vi "FFID_C_Profile.vi"(4 "Traverse line":T1 {"Carrier_2 Q (l/min)" format="%#.2f"; "Row Duration (mins)" format="%#.1f"; "Row No" min=0; "Trace Gas Concentration (%)" min=0.0 format="%#_4f"; "Carrier_1 Q (l/min)" format="%#.4f"; "Start X" format="%#.2f"; "Start Y" format="%#.2f"; "Start Z" format="%#.2f"; "End X" format="%#.2f"; "End Y" format="%#.2f"; "End Z" format="%#.2f"; "Tunnel Speed" format="%#.2f"; "Averaging time (mins)" min=0.0 format="%#.2f"}, 5 "Array of Positions":sgl[][](array[numeric]) format="%.2f", 6 "Loop i":i32, 7 "Arguments":string[](array[string]), 8 "Simulate/Run":T4) -> (0 "Next Position":sgl[](array[numeric]) format="%.2f", 1 "Point index":i32, 2 "Error String":string, 3 "Continue":bool)   [LabVIEW 2022 SP3]
uses:
  Controls/User_Specific_mode.ctl
  Gen Trav/Traverse_cluster.ctl
  Gen Trav/Spacing.ctl
  Controls/Multi_run_mode.ctl
  Controls/Inst_type.ctl
  Globals/Meas_global.vi
panel:
  out "Bad point":bool
  out "Additional Point":dbl[](array[numeric])
  out "Bad Points":i32
  in  "Finished latter part":bool
  out "Positions to visit":sgl[](array[numeric])
  out "Start Postion Used":dbl
  out "Profile                  Max Location":dbl[][](array[numeric])
  out "Index Array":i32[](array[numeric])
  out "First part of Profile":bool=TRUE
  out "Jump":i32
  out "Latter part index":i32
  out "User Start Position":dbl
  out "Threshold":dbl
  out "Cut off %":dbl
  out "New Crossection?":bool
  out "Max value and position":dbl[](array[numeric])
  out "Indexes":i32[](array[numeric])
  out "Crossection Name":string
  out "Current Concentrations":dbl[](array[numeric])
  # "Cmax\n\n\nX  at Cmax\n\nY at Cmax\n\nZ at Cmax\n\n\nXmin\n\nXmax\n\n\nYmin\n\nYmax\n\n\nZmin\n\nZmax"
  # "X           Y          Z"
  # "Start"
  # "End"
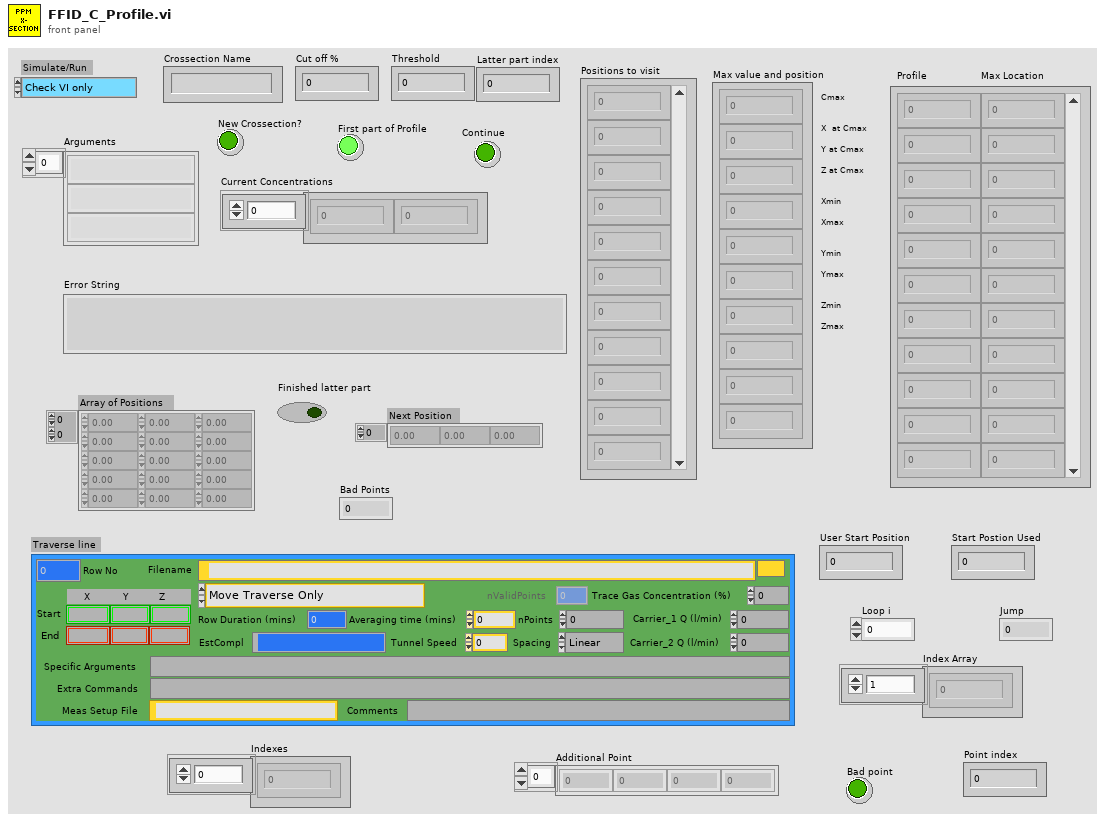
[diagram p1: front panel]
types:
  T1 = typedef "Traverse_cluster.ctl" = cluster{"Start X":sgl, "Start Y":sgl, "Start Z":sgl, "End X":sgl, "End Y":sgl, "End Z":sgl, "nPoints":i32, "Spacing":T2, "Filename":path, "Tunnel Speed":dbl, "Averaging time (mins)":dbl, "Extra Commands":string, "Carrier_1 Q (l/min)":dbl, "Carrier_2 Q (l/min)":dbl, "Trace Gas Concentration (%)":dbl, "Specific Arguments":string, "Comments":string, "Row No":i32, "Row Type Selector":T3, "EstCompl":string, "Row Duration (mins)":dbl, "nValidPoints":i32, "Meas Setup File":string}
  T2 = typedef "Spacing.ctl" = enum16{"Linear", "Log", "Gauss", "Specified", "N/A"}
  T3 = typedef "Multi_run_mode.ctl" = enum16{"Move Traverse Only", "Set Tunnel Speed Only", "Set Source Only", "Set Measurement Conditions", "Single Measurement", "Vertical Profile", "Lateral Profile", "Longitudinal Profile", "Multi-Axis Profile", "Explore Volume", "Auto Calibrate", "Meas Fast FID Bkgnd", "Check Beam Power", "Scanning Valve Measurement", "Run VI Named:", "Set ADAM Ch", "Wait (minutes)", "Send Message", "Synchronize With:", "Fall Back to this Row", "Turn Off Row Repeating", "Traverse 3D Volume", "Blank Row", "Jump to Fall Back Row"}
  T4 = typedef "User_Specific_mode.ctl" = enum16{"Check VI only", "Run VI"}
  T5 = typedef "Inst_type.ctl" = enum16{"Raw voltage", "Raw with zero offsetting", "Propeller anemometer", "Pressure Transducer", "Pitot-static tube", "Hot wire", "Cross wire 1", "Cross wire 2", "Generic Linear", "Generic Polynomial", "Generic BackPoly", "Fast FID", "Thermocouple", "Cold wire", "Pulsed Wire", "LDA Vel", "LDA Tran time", "LDA Arr time", "Microphone"}
  T6 = typedef "Analysis_info_cluster.ctl" = cluster{"Colour":u32, "Inst type":T5, "Inst name":string, "Symbol":string, "Code name":string, "Extra Info":string, "Inst Array":T7, "Extra Titles":string[], "Extra Values":string[], "U":dbl, "u^2":dbl, "u^3":dbl, "u^4":dbl, "Skew_u":dbl, "Kurt_u":dbl, "Sd Error in Mean":dbl, "% u'/U":dbl, "X":dbl, "Y":dbl, "Z":dbl, "Timescale integral Estimate":dbl, "Sd Error in Variance":dbl, "Calib File":path, "Calib Constants":dbl[], "Output Position":bool, "Stats":enum16{"None", "Basic", "Full"}, "Av Sampling Rate":dbl, "Av No of Samples":dbl, "Total Meas Time (s)":dbl, "ADAM Ch Name":string, "Max value":dbl, "Min value":dbl, "Req Sample Rate Hz":dbl, "Sync Delay Time (s)":dbl, "Ch No":i16, "Device":string, "Use Latest Calib":bool, "Port":string, "Metadata Ch Names":string[], "Metadata Ch Values":string[], "Label":string}
  T7 = typedef "Instrument_Array.ctl" = enum16{"PWA", "LDA", "Analogue"}
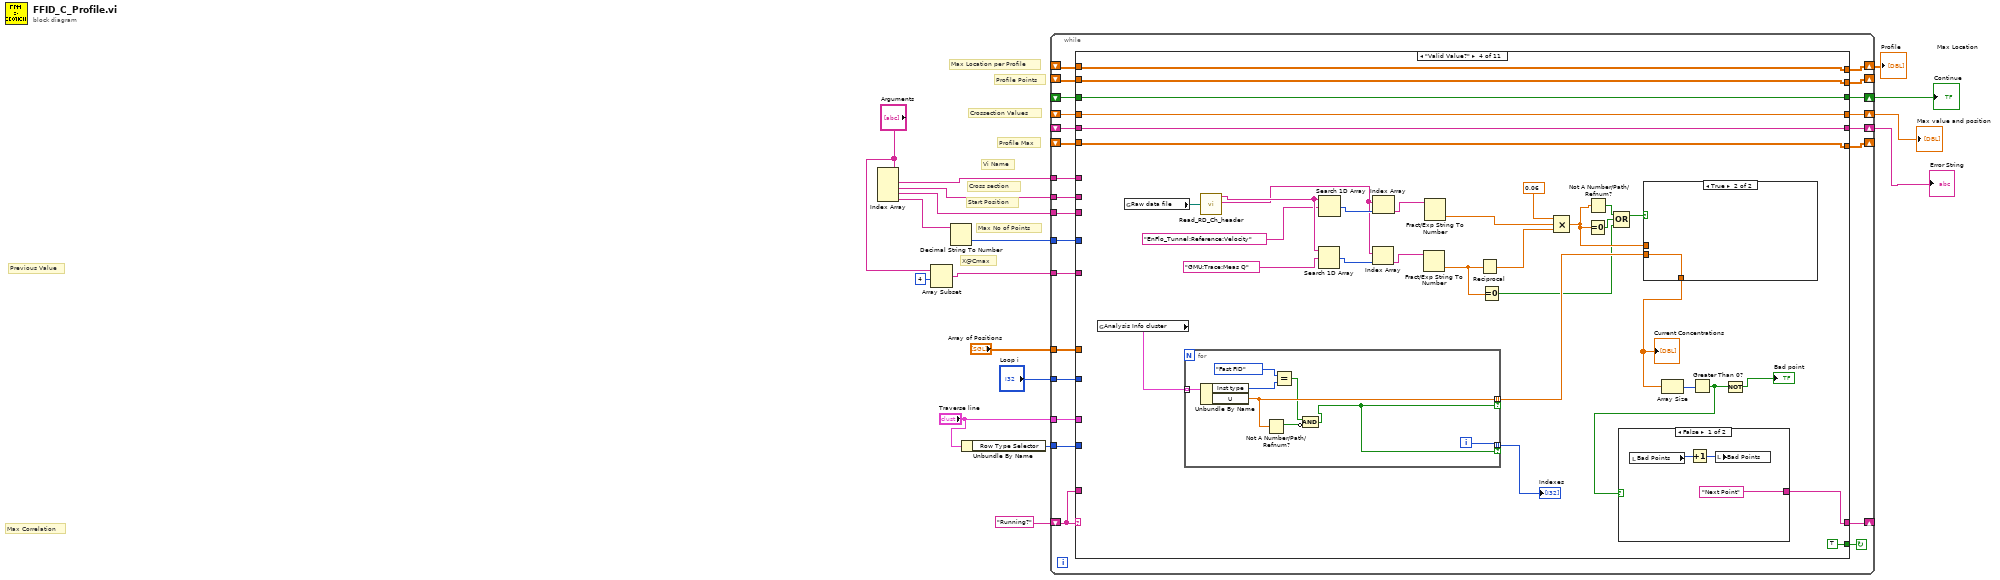
[diagram p0: block diagram]
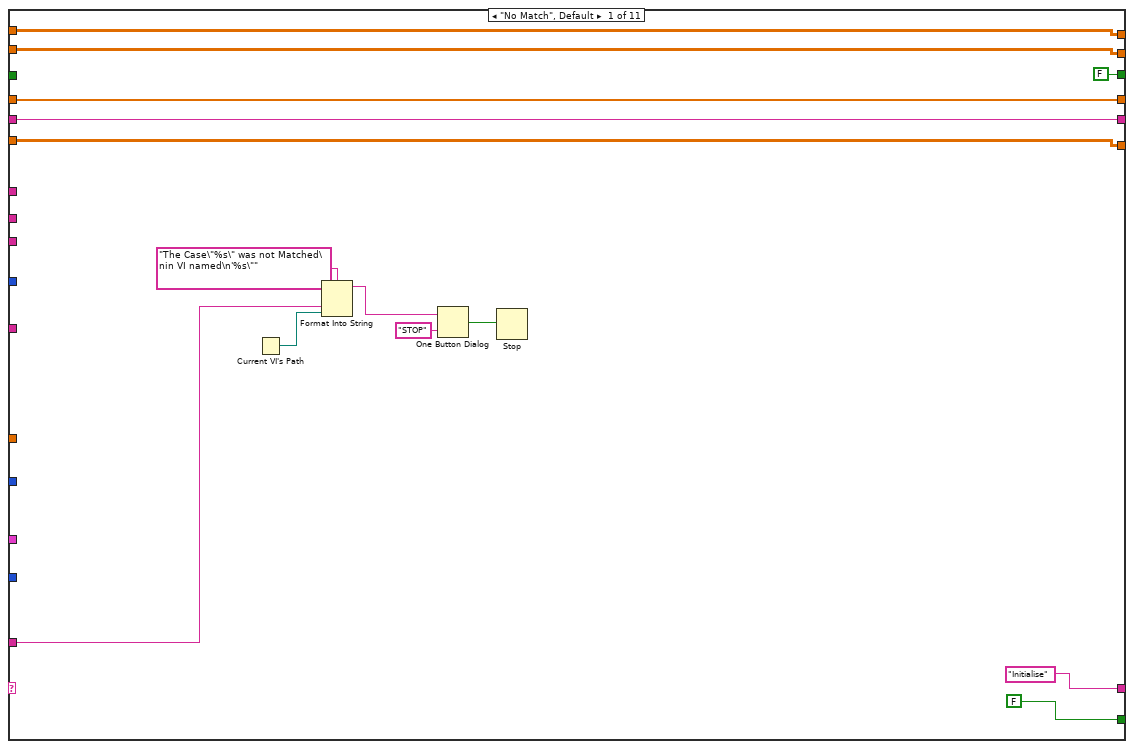
[diagram p2: hidden frame]
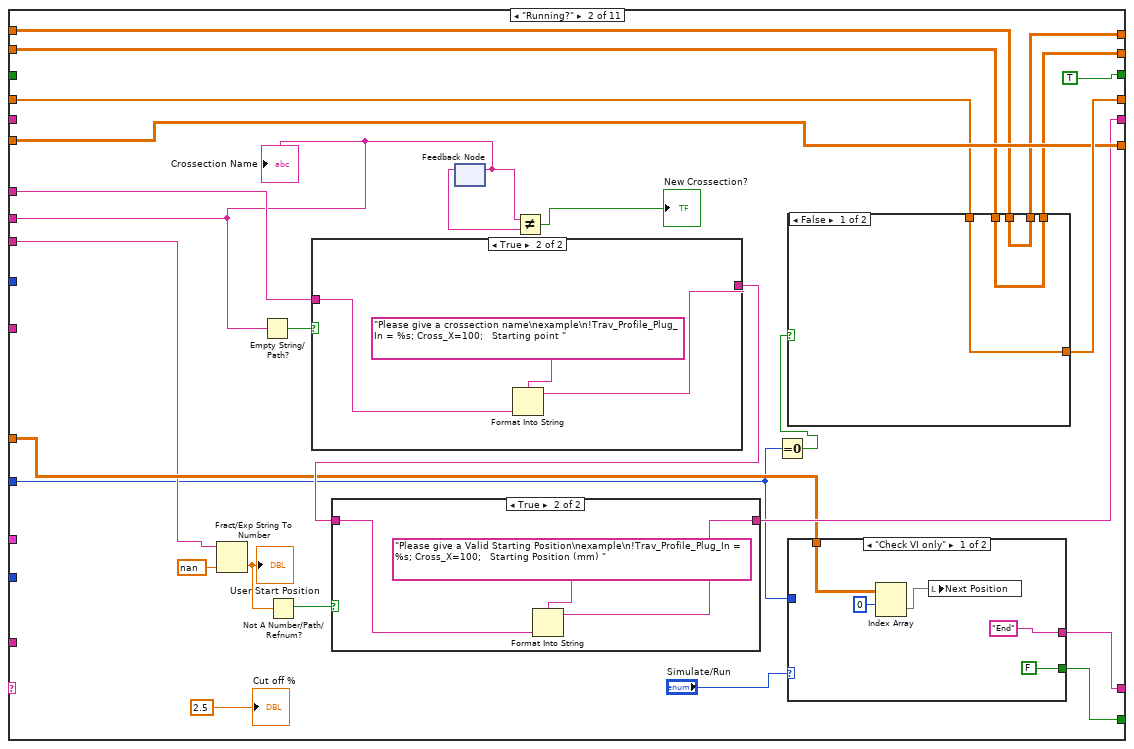
[diagram p3: hidden frame]
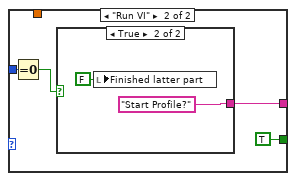
[diagram p4: hidden frame]
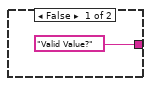
[diagram p5: hidden frame]
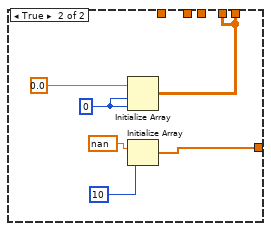
[diagram p7: hidden frame]
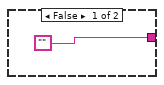
[diagram p8: hidden frame]
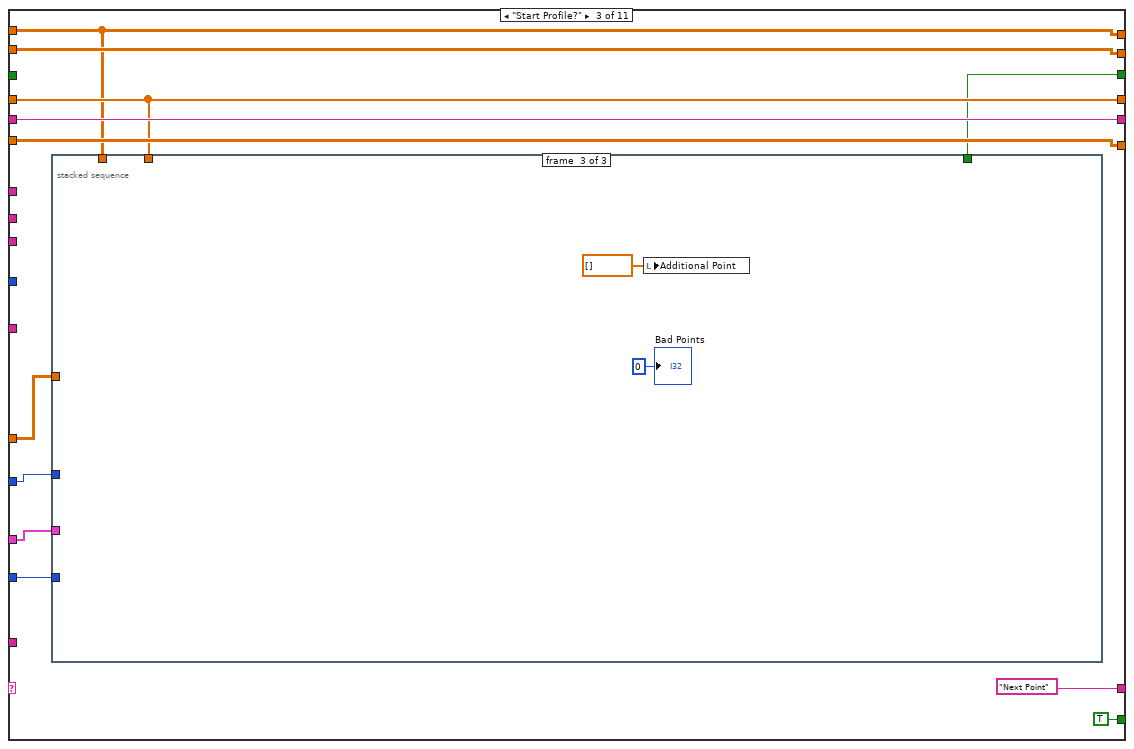
[diagram p9: hidden frame]
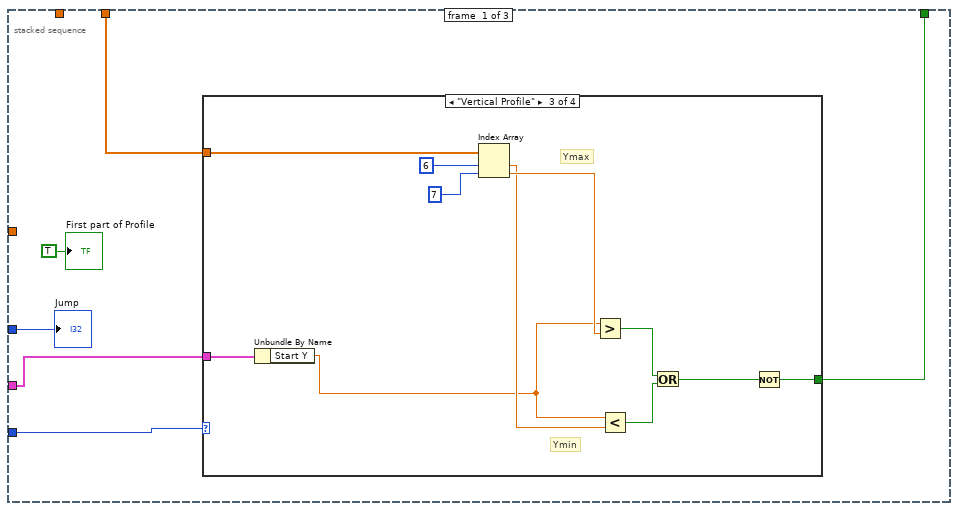
[diagram p10: hidden frame]
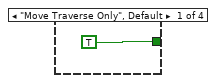
[diagram p11: hidden frame]
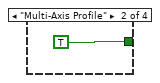
[diagram p12: hidden frame]
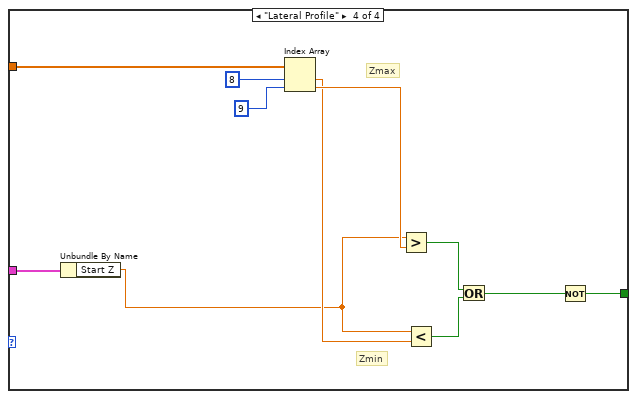
[diagram p13: hidden frame]
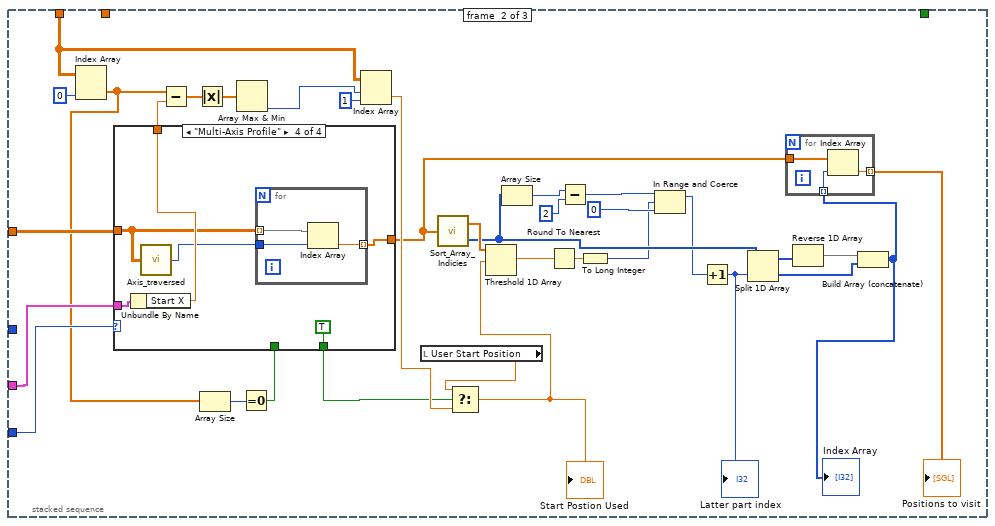
[diagram p14: hidden frame]
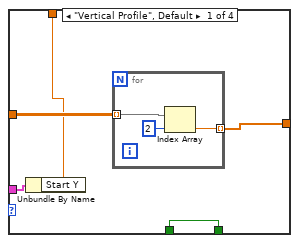
[diagram p15: hidden frame]
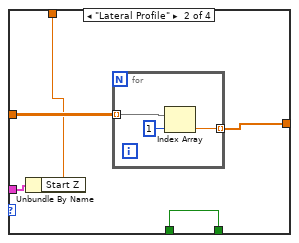
[diagram p16: hidden frame]
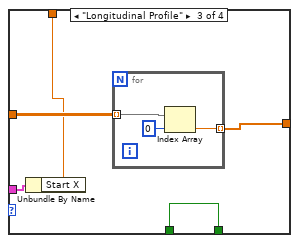
[diagram p17: hidden frame]
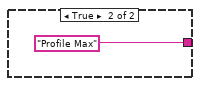
[diagram p18: hidden frame]
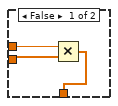
[diagram p19: hidden frame]
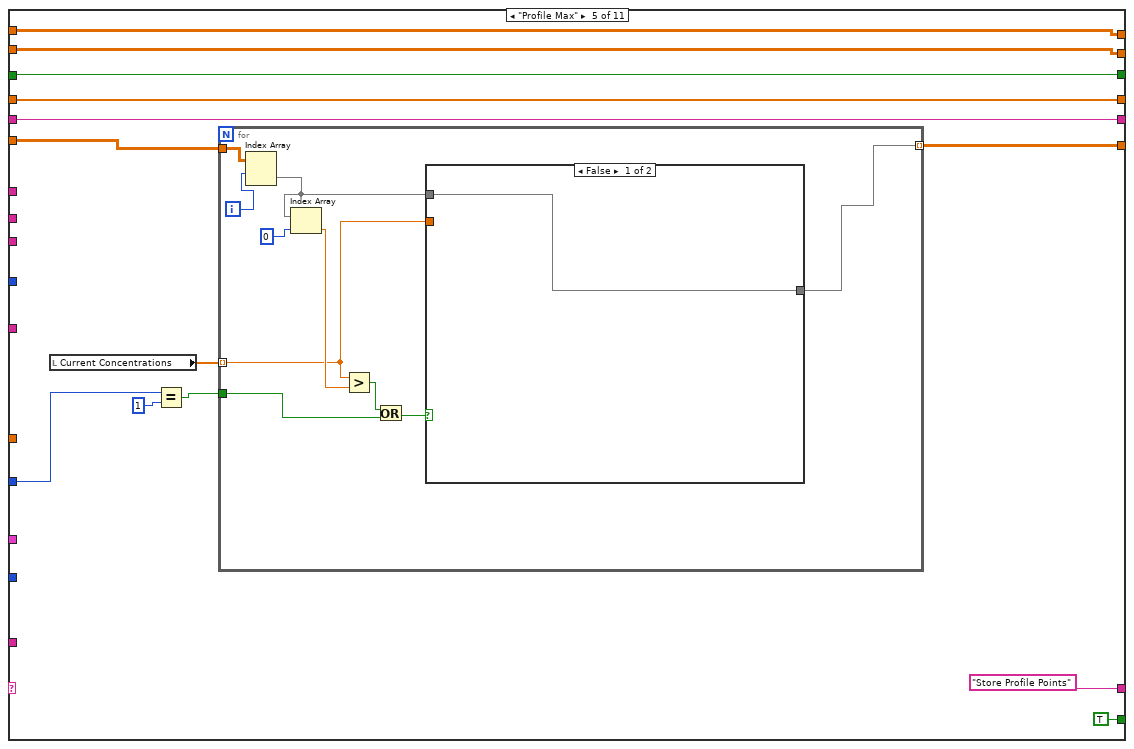
[diagram p20: hidden frame]
diagram:
  # "X@Cmax"
  # "Max No of Points"
  # "Start Position"
  # "Cross section"
  # "Vi Name"
  # "Max Location per Profile"
  # "Profile Points"
  # "Profile Max"
  # "Crossection Values"
  # "Previous Value"
  # "Max Correlation"
  n1 = Index Array(array="Arguments") -> (element #1=w8:string, element #2=w7:string, element #3=w6:string, element #4=w5:string)  [unwired: 4 in]
  n2 = Array Subset(array="Arguments", index=4) -> (w1:string[])  [unwired: 1 in]
  n3 = Decimal String To Number(string=w5) -> (number=w4:i32)  [unwired: 2 in, 1 out]
  n4 = Unbundle By Name("Traverse line") -> ("Row Type Selector"=w11:T3)
  n5 = while {
    shift-left: "Running?" -> [w39]
    shift-right: [w40] -> _
    shift-right: [w38] -> w16
    shift-left: _ -> [w37]
    shift-right: [w36] -> w13
    shift-left: _ -> [w35]
    shift-right: [w34] -> w15
    shift-left: _ -> [w33]
    tunnel: "Loop i" -> [w32]
    shift-right: [w30] -> _
    shift-left: _ -> [w31]
    tunnel: "Traverse line" -> [w29]
    tunnel: w11 -> [w28]
    tunnel: "Array of Positions" -> [w27]
    shift-right: [w26] -> _
    shift-left: _ -> [w25]
    shift-right: [w23] -> w9
    shift-left: _ -> [w24]
    tunnel: w8 -> [w22]
    tunnel: w7 -> [w21]
    tunnel: w6 -> [w20]
    tunnel: w1 -> [w19]
    tunnel: w4 -> [w18]
    stop <- w41 continue-if-true
    n6 = case shown="\"Valid Value?\"" w39 {
      tunnel: [FALSE w63 TRUE TRUE TRUE TRUE TRUE TRUE w471 w504 FALSE] -> w41
      tunnel: ["Initialise" w74 "Next Point" w251 "Store Profile Points" "Cross section Max" w321 "Insert max location" ("t") "Extra Points" ("t") w503 "End"] -> w40
      tunnel: w39 -> [w50 _ _ _ _ _ _ _ _ _ _]
      tunnel: [FALSE TRUE w117 w257 w280 w306 w333 w392 w471 w516 w570] -> w38
      tunnel: w37 -> [_ _ _ w257 w280 w306 _ w392 _ w515 _]
      tunnel: [w46 w77 w118 w256 w281 w307 w342 w387 w474 w513 w572] -> w36
      tunnel: w35 -> [w46 w75 w118 w256 w281 w307 w349 w388 w474 w513 w572]
      tunnel: [w45 w69 w121 w254 w284 w309 w345 w391 w489 w524 w576] -> w34
      tunnel: w33 -> [w45 _ w121 w254 w284 w309 w345 w391 w489 w524 w576]
      tunnel: w32 -> [_ w57 w115 _ w279 _ w329 _ _ w521 w569]
      tunnel: w31 -> [w44 w76 w120 w252 w282 w302 w334 w390 w484 w523 w575]
      tunnel: [w44 w76 w120 w252 w276 w302 w334 w390 w484 w523 w575] -> w30
      tunnel: w29 -> [_ _ w119 _ _ _ _ w383 w481 _ _]
      tunnel: w28 -> [_ _ w113 _ _ _ _ _ w482 _ _]
      tunnel: w27 -> [_ w62 w114 _ _ _ _ _ _ w522 _]
      tunnel: [w43 w67 w112 w249 w275 w304 w331 w381 w487 w506 w557] -> w26
      tunnel: w25 -> [w43 w66 w112 w249 w275 w303 w331 w381 w487 w506 w559]
      tunnel: [w42 w65 w111 w248 w274 w301 w328 w380 w477 w514 w573] -> w23
      tunnel: w24 -> [w42 w64 w111 w248 w274 w301 w328 w380 w476 w514 w573]
      tunnel: w22 -> [_ w61 _ _ _ _ _ _ _ _ _]
      tunnel: w21 -> [_ w60 _ _ _ _ _ _ _ _ _]
      tunnel: w20 -> [_ w59 _ _ _ _ _ _ _ _ _]
      tunnel: w19 -> [_ _ _ _ _ _ w318 _ _ w502 _]
      tunnel: w18 -> [_ _ _ _ _ _ _ _ _ _ w571]
      frame "No Match", Default {
        n7 = Current VI's Path() -> (path=w49:path)
        n8 = Format Into String(format string="The Case\"%s\" was not Matched\nin VI named\n'%s\"" ("Format String"), w50, w49) -> (resulting string=w53:string)  [unwired: 2 in, 1 out]
        n9 = One Button Dialog(message=w53, button name ("OK")="STOP") -> (true=w51:bool)
        n10 = Stop(stop? (T)=w51) -> ()
      }
      frame "Running?" {
        n11 = Fract/Exp String To Number(string=w59, default (0 dbl)=nan ("default (0 DBL)")) -> (number=w72:dbl)  [unwired: 2 in, 1 out]
        "User Start Position" <- w72
        n12 = Empty String/Path?(string/path=w60) -> (empty?=w80:bool)
        n13 = Not A Number/Path/Refnum?(number/path/refnum=w72) -> (NaN/Path/Refnum?=w71:bool)
        n14 = case shown="True" w80 {
          tunnel: ["" w108] -> w70
          tunnel: w61 -> [_ w110]
          frame False {
          }
          frame True {
            n15 = Format Into String(format string="Please give a crossection name\nexample\n!Trav_Profile_Plug_In = %s; Cross_X=100;   Starting point ", w110) -> (resulting string=w108:string)  [unwired: 2 in, 1 out]
          }
        }
        n16 = case shown="True" w71 {
          tunnel: [w94 w95] -> w69
          tunnel: w70 -> [w94 w97]
          frame False {
          }
          frame True {
            n17 = Format Into String(format string="Please give a Valid Starting Position\nexample\n!Trav_Profile_Plug_In = %s; Cross_X=100;   Starting Position (mm) ", w97) -> (resulting string=w95:string)  [unwired: 2 in, 1 out]
          }
        }
        n18 = feedback #1() -> (w79:string)  [unwired: 1 in]
        n19 = feedback-in #1(w60) -> ()
        n20 = Not Equal?(x=w60, y=w79) -> (x != y?=→"New Crossection?":bool)
        n21 = Equal To 0?(x=w57) -> (x = 0?=w56:bool)
        n22 = case shown="False" w56 {
          tunnel: [w100 w104] -> w77
          tunnel: w75 -> [w100 _]
          tunnel: [w99 w101] -> w67
          tunnel: w66 -> [w99 _]
          tunnel: [w98 w101] -> w65
          tunnel: w64 -> [w98 _]
          frame False {
          }
          frame True {
            w102 = 0 ("dimension size")
            n23 = Initialize Array(0.0 ("element"), w102, w102) -> (w101:dbl[][])
            n24 = Initialize Array(nan, 10 ("dimension size")) -> (w104:dbl[])
          }
        }
        n25 = case shown="\"Check VI only\"" "Simulate/Run" {
          tunnel: w57 -> [_ w90]
          tunnel: ["End" ("f") w87] -> w74
          tunnel: [FALSE TRUE] -> w63
          tunnel: w62 -> [w84 _]
          frame "Check VI only" {
            n26 = Index Array(array=w84, index (row)=0) -> (element=w82:sgl[])  [unwired: 1 in]
            n27 = local write "Next Position"(w82) -> ()
          }
          frame "Run VI" {
            n28 = Equal To 0?(x=w90) -> (x = 0?=w88:bool)
            n29 = case shown="True" w88 {
              tunnel: ["Valid Value?" "Start Profile?" ("t")] -> w87
              frame False {
              }
              frame True {
                n30 = local write "Finished latter part"(FALSE ("Finished latter part")) -> ()
              }
            }
          }
        }
        "Crossection Name" <- w60
        "Cut off %" <- 2.5 ("default (0 DBL)")
      }
      frame "Start Profile?" {
        n31 = stacked-sequence {
          tunnel: w119 -> [w123 w184 _]
          tunnel: w118 -> [w128 _ _]
          tunnel: [w127 _ _] -> w117
          tunnel: w115 -> [w126 _ _]
          tunnel: w114 -> [_ w186 _]
          tunnel: w113 -> [w124 w179 _]
          tunnel: w111 -> [_ w183 _]
          frame #0 {
            n32 = case shown="\"Vertical Profile\"" w124 {
              tunnel: w128 -> [_ _ w141 w152]
              tunnel: [TRUE TRUE w140 w151] -> w127
              tunnel: w123 -> [_ _ w132 w143]
              frame "Move Traverse Only", Default {
              }
              frame "Multi-Axis Profile" {
              }
              frame "Vertical Profile" {
                # "Ymax"
                # "Ymin"
                n33 = Unbundle By Name(w132) -> ("Start Y"=w131:sgl)
                n34 = Index Array(array=w141, index #1=6 ("index"), index #2=7 ("index")) -> (element #1=w136:dbl, element #2=w137:dbl)
                n35 = Greater?(x=w131, y=w137) -> (0:w134:bool)
                n36 = Less?(x=w131, y=w136) -> (x < y?=w135:bool)
                n37 = Or(x=w134, y=w135) -> (x .or. y?=w133:bool)
                n38 = Not(x=w133) -> (.not. x?=w140:bool)
              }
              frame "Lateral Profile" {
                # "Zmax"
                # "Zmin"
                n39 = Unbundle By Name(w143) -> ("Start Z"=w142:sgl)
                n40 = Index Array(array=w152, index #1=8 ("index"), index #2=9 ("index")) -> (element #1=w147:dbl, element #2=w148:dbl)
                n41 = Greater?(x=w142, y=w148) -> (0:w145:bool)
                n42 = Less?(x=w142, y=w147) -> (x < y?=w146:bool)
                n43 = Or(x=w145, y=w146) -> (x .or. y?=w144:bool)
                n44 = Not(x=w144) -> (.not. x?=w151:bool)
              }
            }
            "Jump" <- w126
            "First part of Profile" <- TRUE
          }
          frame #1 {
            n45 = Index Array(array=w183, index (col)=0 ("disabled index (col)")) -> (element=w156:dbl[])  [unwired: 1 in]
            n46 = Array Size(array=w156) -> (size(s)=w155:i32)
            n47 = Equal To 0?(x=w155) -> (x = 0?=w153:bool)
            n48 = case shown="\"Multi-Axis Profile\"" w179 {
              tunnel: w186 -> [w194 w202 w210 w216]
              tunnel: [w193 w201 w209 w219] -> w157
              tunnel: w184 -> [w192 w200 w208 w218]
              tunnel: [w191 w199 w207 w217] -> w163
              tunnel: [w190 w198 w206 TRUE] -> w154
              tunnel: w153 -> [w190 w198 w206 _]
              frame "Vertical Profile", Default {
                n49 = Unbundle By Name(w192) -> ("Start Y"=w191:sgl)
                n50 = for {
                  tunnel: w194 -> [w196] mode=indexing
                  tunnel: [w195] -> w193 mode=indexing
                  n51 = Index Array(array=w196, index=2) -> (element=w195:sgl)
                }
              }
              frame "Lateral Profile" {
                n52 = Unbundle By Name(w200) -> ("Start Z"=w199:sgl)
                n53 = for {
                  tunnel: w202 -> [w204] mode=indexing
                  tunnel: [w203] -> w201 mode=indexing
                  n54 = Index Array(array=w204, index=1) -> (element=w203:sgl)
                }
              }
              frame "Longitudinal Profile" {
                n55 = Unbundle By Name(w208) -> ("Start X"=w207:sgl)
                n56 = for {
                  tunnel: w210 -> [w212] mode=indexing
                  tunnel: [w211] -> w209 mode=indexing
                  n57 = Index Array(array=w212, index=0) -> (element=w211:sgl)
                }
              }
              frame "Multi-Axis Profile" {
                n58 = Unbundle By Name(w218) -> ("Start X"=w217:sgl)
                n59 = call "Axis_traversed.vi"("Position array"=w216) -> ("Axis Traversed"=w215:enum16{"X traverse", "Y traverse", "Z traverse"})  [unwired: 4 out]
                n60 = for {
                  tunnel: w216 -> [w222] mode=indexing
                  tunnel: [w221] -> w219 mode=indexing
                  tunnel: w215 -> [w220]
                  n61 = Index Array(array=w222, index=w220) -> (element=w221:sgl)
                }
              }
            }
            n62 = Subtract(x=w156, y=w163) -> (x-y=w162:dbl[])
            n63 = Absolute Value(x=w162) -> (abs(x)=w161:dbl[])
            n64 = Array Max & Min(array=w161) -> (min index (indices)=w159:i32)  [unwired: 3 out]
            n65 = Index Array(array=w183, index (row)=w159, index (col)=1 ("disabled index (col)")) -> (element=w158:dbl)
            n66 = local read "User Start Position"() -> (w172:dbl)
            n67 = call "Sort_Array_Indicies.vi"("unsorted array"=w157) -> ("sorted array"=w178:dbl[], "Sort Index"=w171:i32[])
            n68 = Select(t=w172, s=w154, f=w158) -> (s? t:f=w182:dbl)
            "Start Postion Used" <- w182
            n69 = Threshold 1D Array(2:w182, 3:w178) -> (0:w177:dbl)  [unwired: 1 in]
            n70 = Array Size(array=w171) -> (size(s)=w167:i32)
            n71 = Round To Nearest(number=w177) -> (nearest integer value=w176:dbl)
            n72 = Subtract(x=w167, y=2) -> (x-y=w168:i32)
            n73 = To Long Integer(number=w176) -> (32bit integer=w169:i32)
            n74 = In Range and Coerce(upper limit=w168, x=w169, lower limit=0) -> (coerced(x)=w165:i32)  [unwired: 1 out]
            n75 = Increment(x=w165) -> (x+1=w185:i32)
            "Latter part index" <- w185
            n76 = Split 1D Array(array=w171, index=w185) -> (first subarray=w175:i32[], second subarray=w173:i32[])
            n77 = Reverse 1D Array(array=w175) -> (reversed array=w174:i32[])
            n78 = Build Array (concatenate)(w174, w173) -> (w181:i32[])
            "Index Array" <- w181
            n79 = for {
              tunnel: w181 -> [w189] mode=indexing
              tunnel: w157 -> [w188]
              tunnel: [w187] -> w180 mode=indexing
              n80 = Index Array(array=w188, index=w189) -> (element=w187:sgl)
            }
            "Positions to visit" <- w180
          }
          frame #2 {
            n81 = local write "Additional Point"(dbl[] [] ("Additional Point")) -> ()
            "Bad Points" <- 0 ("Bad Points")
          }
        }
      }
      frame "Valid Value?" {
        n82 = global read "Meas_global.vi" "Analysis Info cluster"() -> (w247:T6[])
        n83 = global read "Meas_global.vi" "Raw data file"() -> (w246:path)
        n84 = for {
          tunnel: w247 -> [w273] mode=indexing
          tunnel: [w270] -> w230 mode=indexing if=w266
          tunnel: [w267] -> w253 mode=indexing if=w266
          i -> [w267]
          n85 = Unbundle By Name(w273) -> ("Inst type"=w272:T5, "U"=w270:dbl)
          n86 = Not A Number/Path/Refnum?(number/path/refnum=w270) -> (NaN/Path/Refnum?=w269:bool)
          n87 = Equal?(x=Inst_type."Fast FID" ("Inst type"), y=w272) -> (x = y?=w268:bool)
          n88 = Compound Arithmetic op=AND(w268, invert w269) -> (w266:bool)
        }
        "Indexes" <- w253
        n89 = call "Read_RD_Ch_header.vi"("Raw data file"=w246) -> ("Ch Name Out"=w241:string[], "Ch Values"=w240:string[])  [unwired: 2 out]
        n90 = Search 1D Array(1D array=w241, element="GMU:Trace:Meas Q") -> (index of element=w242:i32)  [unwired: 1 in]
        n91 = Search 1D Array(1D array=w241, element="EnFlo_Tunnel:Reference:Velocity") -> (index of element=w245:i32)  [unwired: 1 in]
        n92 = Index Array(array=w240, index=w242) -> (element=w243:string)
        n93 = Index Array(array=w240, index=w245) -> (element=w244:string)
        n94 = Fract/Exp String To Number(string=w243) -> (number=w228:dbl)  [unwired: 3 in, 1 out]
        n95 = Fract/Exp String To Number(string=w244) -> (number=w235:dbl)  [unwired: 3 in, 1 out]
        n96 = Reciprocal(x=w228) -> (1/x=w236:dbl)
        n97 = Equal To 0?(x=w228) -> (x = 0?=w227:bool)
        n98 = Compound Arithmetic op=MULTIPLY(0.06 ("value"), w235, w236) -> (w229:dbl)
        n99 = Equal To 0?(x=w229) -> (x = 0?=w234:bool)
        n100 = Not A Number/Path/Refnum?(number/path/refnum=w229) -> (NaN/Path/Refnum?=w233:bool)
        n101 = Compound Arithmetic op=OR(w233, w234, w227) -> (w232:bool)
        n102 = case shown="True" w232 {
          tunnel: [w262 w265] -> w231
          tunnel: w230 -> [w264 w265]
          tunnel: w229 -> [w263 _]
          frame False {
            n103 = Multiply(x=w263, y=w264) -> (x*y=w262:dbl[])
          }
          frame True {
          }
        }
        "Current Concentrations" <- w231
        n104 = Array Size(array=w231) -> (size(s)=w255:i32)
        n105 = Greater Than 0?(x=w255) -> (x > 0?=w226:bool)
        n106 = case shown="False" w226 {
          tunnel: ["Next Point" ("f") "Profile Max"] -> w251
          frame False {
            n107 = local read "Bad Points"() -> (w259:i32)
            n108 = Increment(x=w259) -> (x+1=w258:i32)
            n109 = local write "Bad Points"(w258) -> ()
          }
          frame True {
          }
        }
        n110 = Not(x=w226) -> (.not. x?=→"Bad point":bool)
      }
      frame "Profile Max" {
        n111 = local read "Current Concentrations"() -> (w283:dbl[])
        n112 = Equal?(x=w279, y=1) -> (x = y?=w277:bool)
        n113 = for {
          tunnel: w283 -> [w294] mode=indexing
          tunnel: w277 -> [w292]
          tunnel: w282 -> [w289]
          tunnel: [w291] -> w276 mode=indexing
          i -> [w290]
          n114 = Index Array(array=w289, index (row)=w290) -> (element=w288:dbl[])  [unwired: 1 in]
          n115 = Index Array(array=w288, index=0) -> (element=w296:dbl)
          n116 = Greater?(x=w294, y=w296) -> (0:w293:bool)
          n117 = Or(x=w293, y=w292) -> (x .or. y?=w295:bool)
          n118 = case shown="False" w295 {
            tunnel: w294 -> [_ w300]
            tunnel: [w297 w299] -> w291
            tunnel: w288 -> [w297 _]
            frame False {
            }
            frame True {
              n119 = local read "Next Position"() -> (w298:sgl[])
              n120 = Build Array (concatenate)(w300, w298) -> (w299:dbl[])
            }
          }
        }
      }
      frame "Store Profile Points" {
        n121 = local read "Current Concentrations"() -> (w308:dbl[])
        n122 = for {
          tunnel: w308 -> [w314] mode=indexing
          tunnel: [w313] -> w305 mode=indexing
          n123 = local read "Next Position"() -> (w312:sgl[])
          n124 = Build Array (concatenate)(w312, w314) -> (w313:dbl[])
        }
        n125 = Build Array (concatenate)(w303, w305) -> (w304:dbl[][])
      }
      frame "Cross section Max" {
        n126 = Array Size(array=w318) -> (size(s)=w317:i32)
        n127 = local read "Current Concentrations"() -> (w350:dbl[])
        n128 = Equal To 0?(x=w317) -> (x = 0?=w316:bool)
        n129 = Array Max & Min(array=w350) -> (max value=w346:dbl, max index (indices)=w344:i32)  [unwired: 2 out]
        n130 = local read "Cut off %"() -> (w340:dbl)
        n131 = Index Array(array=w349, index=0) -> (element=w338:dbl)
        n132 = Not A Number/Path/Refnum?(number/path/refnum=w338) -> (NaN/Path/Refnum?=w336:bool)
        n133 = local read "New Crossection?"() -> (w324:bool)
        n134 = Greater?(x=w346, y=w338) -> (0:w337:bool)
        n135 = Or(x=w336, y=w337) -> (x .or. y?=w335:bool)
        n136 = case shown="True" w335 {
          tunnel: w344 -> [_ _]
          tunnel: w346 -> [_ w378]
          tunnel: [w372 w377] -> w342
          tunnel: w349 -> [w372 w376]
          frame False {
          }
          frame True {
            n137 = local read "Next Position"() -> (w373:sgl[])
            n138 = Array Subset(array=w376, index=4) -> (w374:dbl[])  [unwired: 1 in]
            n139 = Build Array (concatenate)(w378, w373, w374) -> (w377:dbl[])
          }
        }
        n140 = Divide(x=w340, y=100.0) -> (x/y=w347:dbl)
        n141 = Index Array(array=w342, index=0) -> (element=w341:dbl)
        n142 = Multiply(x=w341, y=w347) -> (x*y=w323:dbl)
        n143 = case shown="True" w324 {
          tunnel: [w353 w355] -> w315
          tunnel: w323 -> [w354 w355]
          frame False {
            n144 = In Range and Coerce(upper limit=4.0, x=w354, lower limit=0.01) -> (coerced(x)=w353:dbl)  [unwired: 1 out]
          }
          frame True {
          }
        }
        "Threshold" <- w315
        n145 = Greater?(x=w346, y=w315) -> (0:w327:bool)
        n146 = local read "First part of Profile"() -> (w330:bool)
        n147 = Select(t=w327, s=w316, f=TRUE) -> (s? t:f=w326:bool)
        n148 = case shown="True" w330 {
          tunnel: [w356 TRUE] -> w333
          tunnel: w329 -> [_ w366]
          tunnel: w326 -> [w356 w361]
          tunnel: [w357 "Next Point" ("f")] -> w322
          tunnel: w329 -> [_ w364]
          frame False {
            n149 = case shown="False" w356 {
              tunnel: ["Insert limits" "Next Point" ("f")] -> w357
              frame False {
              }
              frame True {
              }
            }
          }
          frame True {
            n150 = local read "Latter part index"() -> (w363:i32)
            n151 = Less?(x=w364, y=w363) -> (x < y?=w362:bool)
            n152 = And(x=w362, y=w361) -> (x .and. y?=w360:bool)
            n153 = case shown="False" w360 {
              tunnel: w366 -> [w371 _]
              tunnel: w363 -> [w368 _]
              frame False {
                n154 = local write "First part of Profile"(FALSE) -> ()
                n155 = Subtract(x=w368, y=w371) -> (x-y=w370:i32)
                n156 = local write "Jump"(w370) -> ()
              }
              frame True {
              }
            }
          }
        }
        n157 = Select(t="Extra Points", s="Finished latter part", f=w322) -> (s? t:f=w321:string)
      }
      frame "Insert limits" {
        n158 = Unbundle By Name(w383) -> ("Row Type Selector"=w384:T3, "Start Y"=w382:sgl, "Start Z"=w379:sgl)
        n159 = local read "Threshold"() -> (w389:dbl)
        n160 = for {
          tunnel: w390 -> [w397] mode=indexing
          tunnel: w389 -> [w400]
          tunnel: w384 -> [w398]
          shift-right: [w395] -> w387
          shift-left: w388 -> [w396]
          tunnel: w382 -> [w394]
          tunnel: w379 -> [w393]
          n161 = Index Array(array=w397, index=0) -> (element=w401:dbl)
          n162 = Greater?(x=w401, y=w400) -> (0:w399:bool)
          n163 = case shown="False" w399 {
            tunnel: w398 -> [w408 _]
            tunnel: w396 -> [w407 w470]
            tunnel: w397 -> [w406 _]
            tunnel: [w405 w470] -> w395
            tunnel: w394 -> [w404 _]
            tunnel: w393 -> [w403 _]
            frame False {
              n164 = case shown="\"Lateral Profile\"" w408 {
                tunnel: w407 -> [w409 w412 w442]
                tunnel: w406 -> [_ _ _]
                tunnel: [w409 w411 w441] -> w405
                tunnel: w404 -> [_ w410 _]
                tunnel: w403 -> [_ _ w440]
                frame "Move Traverse Only", Default {
                }
                frame "Vertical Profile" {
                  n165 = Index Array(array=w412, index=2) -> (element=w414:dbl)
                  n166 = Greater?(x=w410, y=w414) -> (0:w413:bool)
                  n167 = case shown="False" w413 {
                    tunnel: w412 -> [w419 w431]
                    tunnel: w410 -> [w417 w429]
                    tunnel: [w416 w428] -> w411
                    frame True {
                      # "Ymax"
                      n168 = in-place {
                        in-place-border: w417 -> [w421]
                        n169 = in-place-array #2(w419, 7) -> (w420:dbl)
                        n170 = Not A Number/Path/Refnum?(number/path/refnum=w420) -> (NaN/Path/Refnum?=w423:bool)
                        n171 = case shown="False" w423 {
                          tunnel: [w424 w427] -> w422
                          tunnel: w421 -> [w426 w427]
                          tunnel: w420 -> [w425 _]
                          frame False {
                            n172 = Max & Min(x=w425, y=w426) -> (min(x,y)=w424:dbl)  [unwired: 1 out]
                          }
                          frame True {
                          }
                        }
                        n173 = in-place-array #2(w422) -> (w416:dbl[])  [unwired: 1 out]
                      }
                    }
                    frame False {
                      # "Ymin"
                      n174 = in-place {
                        in-place-border: w429 -> [w433]
                        n175 = in-place-array #3(w431, 6) -> (w432:dbl)
                        n176 = Not A Number/Path/Refnum?(number/path/refnum=w432) -> (NaN/Path/Refnum?=w435:bool)
                        n177 = case shown="False" w435 {
                          tunnel: [w436 w439] -> w434
                          tunnel: w433 -> [w438 w439]
                          tunnel: w432 -> [w437 _]
                          frame False {
                            n178 = Max & Min(x=w437, y=w438) -> (max(x,y)=w436:dbl)  [unwired: 1 out]
                          }
                          frame True {
                          }
                        }
                        n179 = in-place-array #3(w434) -> (w428:dbl[])  [unwired: 1 out]
                      }
                    }
                  }
                }
                frame "Lateral Profile" {
                  n180 = Index Array(array=w442, index=3) -> (element=w444:dbl)
                  n181 = Greater?(x=w440, y=w444) -> (0:w443:bool)
                  n182 = case shown="False" w443 {
                    tunnel: w442 -> [w449 w461]
                    tunnel: w440 -> [w447 w459]
                    tunnel: [w446 w458] -> w441
                    frame True {
                      # "Zmax"
                      n183 = in-place {
                        in-place-border: w447 -> [w451]
                        n184 = in-place-array #4(w449, 9) -> (w450:dbl)
                        n185 = Not A Number/Path/Refnum?(number/path/refnum=w450) -> (NaN/Path/Refnum?=w453:bool)
                        n186 = case shown="False" w453 {
                          tunnel: [w454 w457] -> w452
                          tunnel: w451 -> [w456 w457]
                          tunnel: w450 -> [w455 _]
                          frame False {
                            n187 = Max & Min(x=w455, y=w456) -> (min(x,y)=w454:dbl)  [unwired: 1 out]
                          }
                          frame True {
                          }
                        }
                        n188 = in-place-array #4(w452) -> (w446:dbl[])  [unwired: 1 out]
                      }
                    }
                    frame False {
                      # "Zmin"
                      n189 = in-place {
                        in-place-border: w459 -> [w463]
                        n190 = in-place-array #5(w461, 8) -> (w462:dbl)
                        n191 = Not A Number/Path/Refnum?(number/path/refnum=w462) -> (NaN/Path/Refnum?=w465:bool)
                        n192 = case shown="False" w465 {
                          tunnel: [w466 w469] -> w464
                          tunnel: w463 -> [w468 w469]
                          tunnel: w462 -> [w467 _]
                          frame False {
                            n193 = Max & Min(x=w467, y=w468) -> (max(x,y)=w466:dbl)  [unwired: 1 out]
                          }
                          frame True {
                          }
                        }
                        n194 = in-place-array #5(w464) -> (w458:dbl[])  [unwired: 1 out]
                      }
                    }
                  }
                }
              }
            }
            frame True {
            }
          }
        }
      }
      frame "Insert max location" {
        w472 = 0.1  # Cmax must be greater than this to add extra points
        n195 = for {
          tunnel: w484 -> [w497] mode=indexing
          tunnel: [w496] -> w486 mode=indexing
          n196 = Index Array(array=w497, index=0) -> (element=w496:dbl)
        }
        n197 = case shown="\"Lateral Profile\"" w482 {
          tunnel: [3 ("max index(es)") 2 ("max index(es)")] -> w483
          tunnel: w481 -> [w491 w494]
          tunnel: [w490 w493] -> w480
          frame "Vertical Profile", Default {
            n198 = Unbundle By Name(w491) -> ("Start Y"=w490:sgl)
          }
          frame "Lateral Profile" {
            n199 = Unbundle By Name(w494) -> ("Start Z"=w493:sgl)
          }
        }
        n200 = Array Max & Min(array=w486) -> (max index (indices)=w485:i32)  [unwired: 3 out]
        n201 = Index Array(array=w484, index (row)=w485, index (col)=w483) -> (element=w479:dbl)
        n202 = Build Array(w480, w479) -> (w478:dbl[])
        n203 = Index Array(array=w474) -> (element=w473:dbl)  [unwired: 1 in]
        n204 = Greater?(x=w473, y=w472) -> (0:w471:bool)
        n205 = local write "Finished latter part"(TRUE ("Finished latter part")) -> ()
        n206 = Build Array (concatenate)(w476, w478) -> (w477:dbl[][])
      }
      frame "Next Point" {
        n207 = local read "Jump"() -> (w500:i32)
        n208 = Greater Than 0?(x=w500) -> (x > 0?=w499:bool)
        n209 = case shown="False" w499 {
          tunnel: w521 -> [w525 w528]
          tunnel: [w525 w527] -> w519
          tunnel: w500 -> [_ w526]
          frame False {
          }
          frame True {
            n210 = Add(x=w528, y=w526) -> (x+y=w527:i32)
          }
        }
        n211 = To Upper Case(1:w502) -> (0:w507:string[])
        n212 = Build Array("X@Cmax" ("element"), "Y@Cmax" ("element"), "Z@Cmax" ("element")) -> (w508:string[])
        n213 = local read "Index Array"() -> (w520:i32[])
        n214 = Array Size(array=w520) -> (size(s)=w518:i32)
        n215 = Index Array(array=w520, index=w519) -> (element=w501:i32)
        "Point index" <- w501
        n216 = Less?(x=w519, y=w518) -> (x < y?=w517:bool)
        n217 = Index Array(array=w522, index (row)=w501) -> (element=w512:sgl[])  [unwired: 1 in]
        n218 = for {
          tunnel: w513 -> [w536]
          shift-right: [w532] -> w505
          shift-left: w512 -> [w531]
          tunnel: w507 -> [w535]
          tunnel: w508 -> [w534] mode=indexing
          i -> [w530]
          n219 = To Upper Case(1:w534) -> (0:w529:string)
          n220 = Search 1D Array(1D array=w535, element=w529) -> (index of element=w533:i32)  [unwired: 1 in]
          n221 = case shown="-1" w533 {
            tunnel: w536 -> [_ w543]
            tunnel: [w537 w541] -> w532
            tunnel: w531 -> [w537 w542]
            tunnel: w530 -> [_ w539]
            frame -1 {
            }
            frame Default {
              n222 = Increment(x=w539) -> (x+1=w540:i32)
              n223 = Index Array(array=w543, index=w540) -> (element=w538:dbl)
              n224 = Replace Array Subset(array=w542, new element=w538, index=w539) -> (w541:sgl[])
            }
          }
        }
        "Next Position" <- w505
        n225 = case shown="True" w517 {
          tunnel: [FALSE ("Continue?") w547] -> w516
          tunnel: w515 -> [_ w548]
          tunnel: [TRUE w549] -> w504
          tunnel: ["Extra Points" w550] -> w503
          frame False {
          }
          frame True {
            n226 = case shown="True" w548 {
              selector: w548 -> [_ w554]
              tunnel: ["Extra Points" ("t") "End"] -> w550
              tunnel: [TRUE FALSE] -> w549
              tunnel: [FALSE w554] -> w547
              frame False {
              }
              frame True {
              }
            }
          }
        }
      }
      frame "Extra Points" {
        n227 = local read "Bad Points"() -> (w568:i32)
        n228 = local read "Additional Point"() -> (w558:dbl[])
        n229 = Subtract(x=w569, y=w568) -> (x-y=w567:i32)
        n230 = local read "Bad point"() -> (w562:bool)
        n231 = Array Size(array=w558) -> (size(s)=w563:i32)
        n232 = Greater Than 0?(x=w563) -> (x > 0?=w561:bool)
        n233 = And(x=w562, y=w561) -> (x .and. y?=w560:bool)
        n234 = Less?(x=w567, y=w571) -> (x < y?=w570:bool)
        n235 = case shown="True" w560 {
          tunnel: w559 -> [w578 w581]
          tunnel: w558 -> [_ w580]
          tunnel: [w578 w579] -> w557
          frame False {
          }
          frame True {
            n236 = Build Array (concatenate)(w581, w580) -> (w579:dbl[][])
          }
        }
        n237 = call "Add Extra position.vi"("Positions"=w557) -> ("Additional Point"=w566:dbl[])  [unwired: 3 in]
        "Additional Point" <- w566
        n238 = Array Subset(array=w566, length=3) -> (w564:dbl[])  [unwired: 1 in]
        n239 = local write "Next Position"(w564) -> ()
      }
    }
  }
  "Continue" <- w16
  "Error String" <- w15
  "Max value and position" <- w13
  "Profile                  Max Location" <- w9
